vi "Read Port.vi"(8 "error in (no error)":errorcluster, 11 "BuildWorker in":refnum<class "BuildWorker.lvclass">) -> (0 "error out":errorcluster, 2 "Port":u16, 3 "BuildWorker out":refnum<class "BuildWorker.lvclass">)   [LabVIEW 2017, in "BuildWorker Interface.lvlib" / "BuildWorker.lvclass"]
uses:
  BuildWorker.lvclass
  BuildWorker.lvclass/BuildWorker.ctl
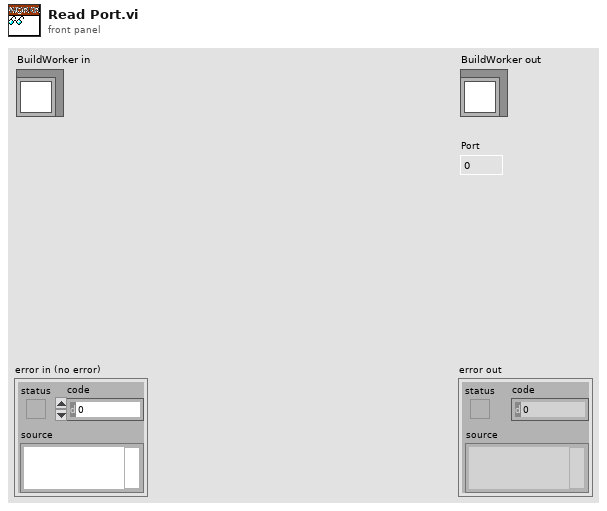
[diagram p1: front panel]
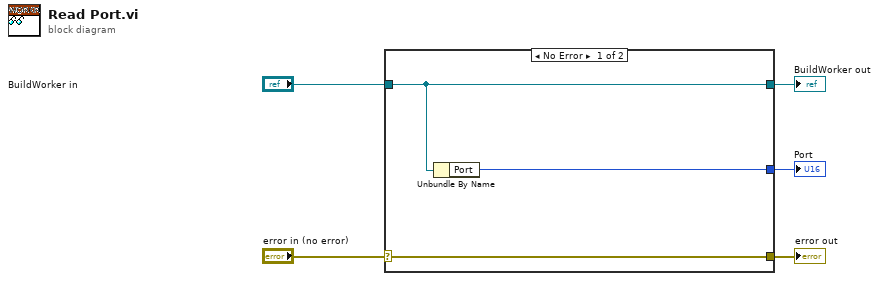
[diagram p0: block diagram]
diagram:
  n1 = case shown="No Error" "error in (no error)" {
    selector: "error in (no error)" -> [w8 w9]
    tunnel: [w8 w9] -> w4
    tunnel: [w7 w10] -> w2
    tunnel: "BuildWorker in" -> [w7 w10]
    tunnel: [w6 _] -> w1
    frame No Error {
      n2 = Unbundle By Name(w7) -> ("Port"=w6:u16)
    }
    frame Error {
    }
  }
  "error out" <- w4
  "BuildWorker out" <- w2
  "Port" <- w1
